vi "Sub Process.vi"(8 "error in (no error)":errorcluster, 11 "MPC_Laser Marked in":refnum<class "MPC_Laser Marked.lvclass">) -> (0 "error out":errorcluster, 3 "MPC_Laser Marked out":refnum<class "MPC_Laser Marked.lvclass">)   [LabVIEW 2019, in "MPC_Laser Marked.lvclass"]
uses:
  MPC_Laser Marked.lvclass
  Main Process Class VI/Ctrl/Flow Action Name.ctl
  Glb/Flow Imform.vi
  LLB/Commonly VI.lvlib
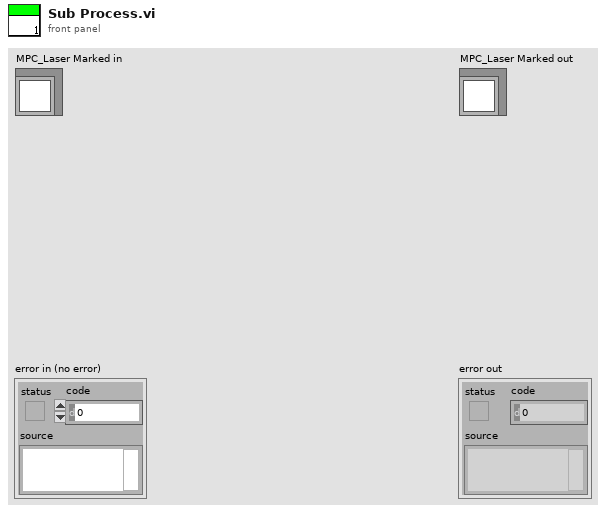
[diagram p1: front panel]
types:
  T1 = typedef "Flow Action Name.ctl" = enum16{"request board", "wait board in", "transfer board in", "imform robot action", "wait robot imform out", "Close Imform Robot", "imform ready out", "wait request", "flow out"}
  T2 = cluster{"AutoRunFlg":refnum<vi>, "Action Finish Flg":refnum<vi>, "Remaining Action":refnum<vi>, "Btn_AutoRun":refnum<vi>, "Manual Flg":refnum<vi>, "Sub Process Error":refnum<vi>}
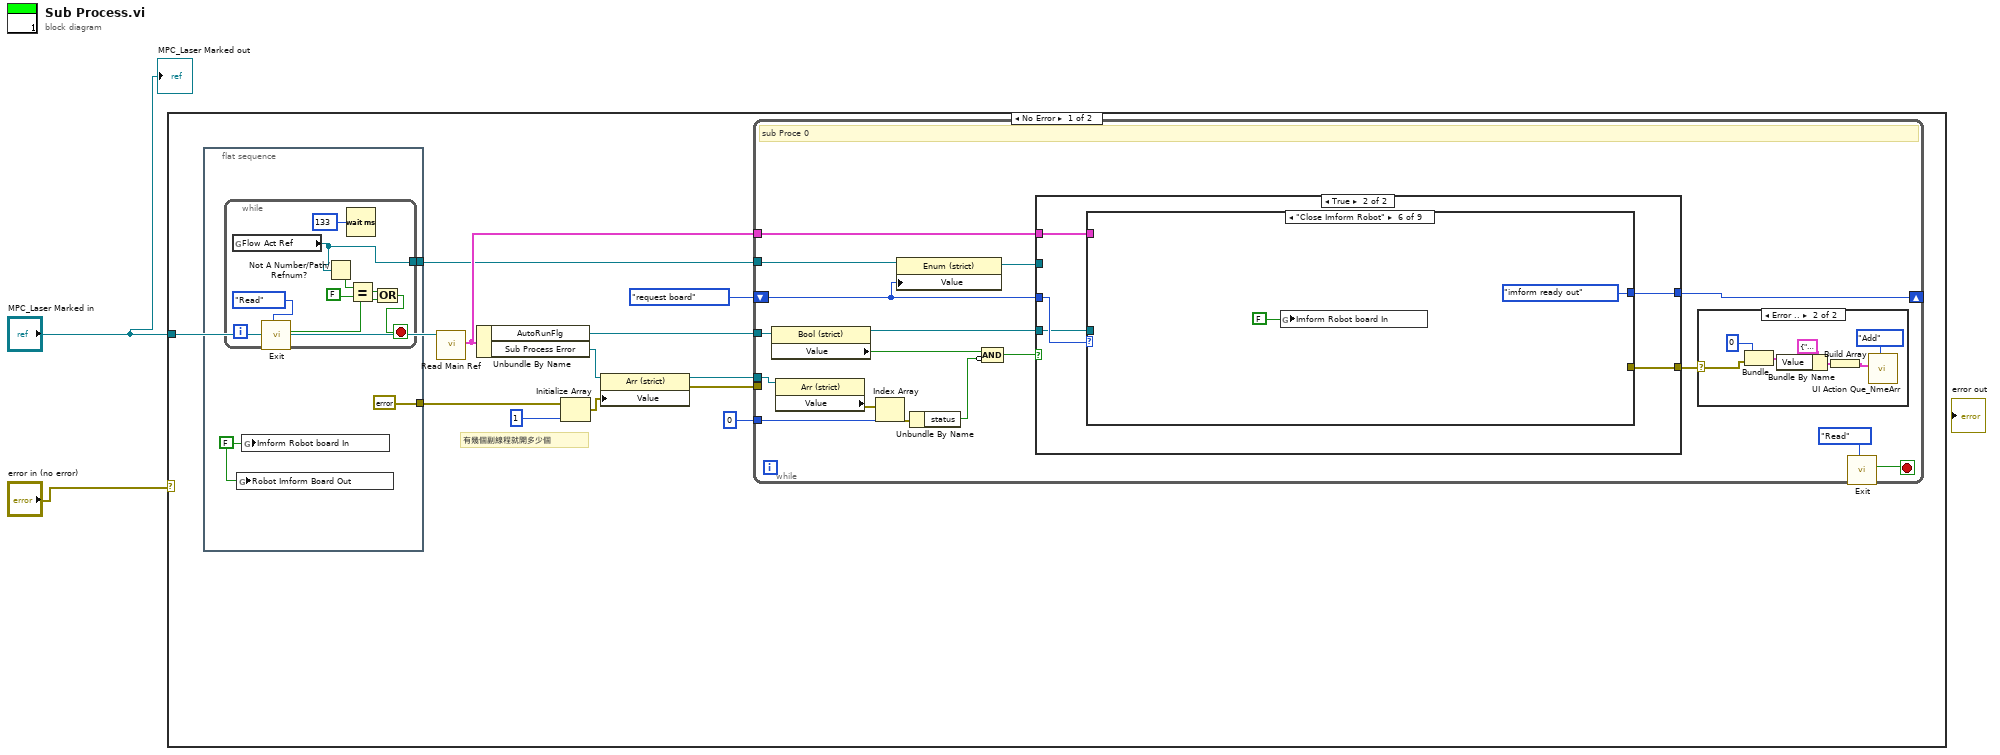
[diagram p0: block diagram]
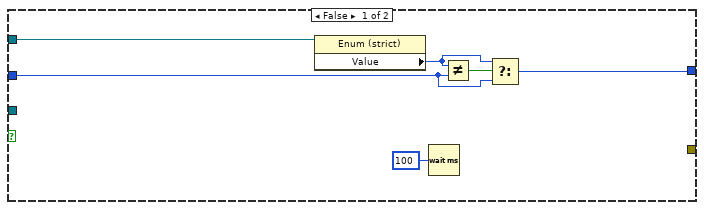
[diagram p3: hidden frame]
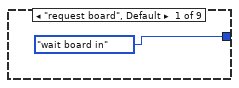
[diagram p4: hidden frame]
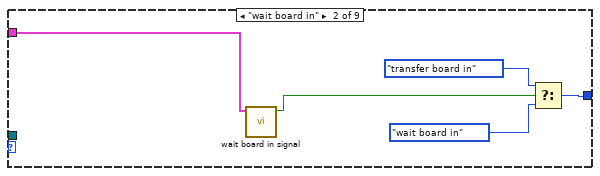
[diagram p5: hidden frame]
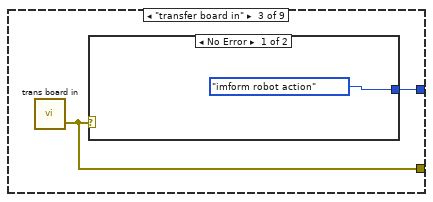
[diagram p6: hidden frame]
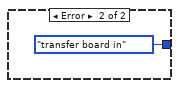
[diagram p7: hidden frame]
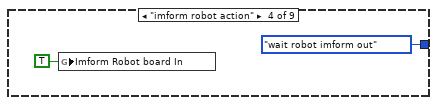
[diagram p8: hidden frame]
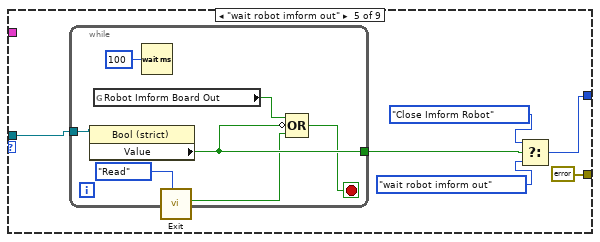
[diagram p9: hidden frame]
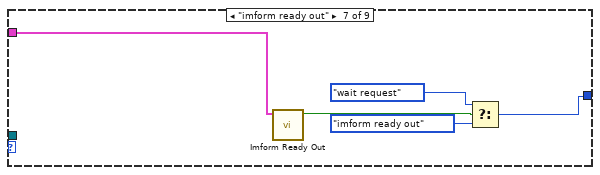
[diagram p10: hidden frame]
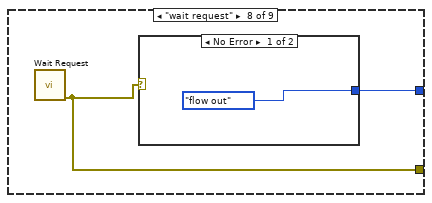
[diagram p11: hidden frame]
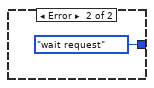
[diagram p12: hidden frame]
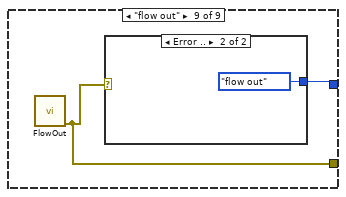
[diagram p13: hidden frame]
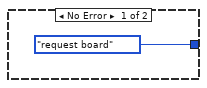
[diagram p14: hidden frame]
diagram:
  n1 = case shown="No Error" "error in (no error)" {
    tunnel: "MPC_Laser Marked in" -> [w14 _]
    frame No Error {
      # "有幾個副線程就開多少個"
      n2 = flat-sequence {
        tunnel: [errorcluster {"status"=FALSE, "code"=0, "source"=""} ("error")] -> w4
        tunnel: [w15] -> w3
        frame #0 {
          w16 = FALSE ("Imform Robot board In")
          n3 = while {
            tunnel: [w24] -> w15
            stop <- w19 stop-if-true
            n4 = global read "Flow Imform.vi" "Flow Act Ref"() -> (w24:refnum<vi>)
            n5 = call "Exit.vi"("Enum"=enum16{"Initial", "Read", "Write"}."Read") -> ("ExitOut"=w20:bool)  [unwired: 10 in]
            n6 = Not A Number/Path/Refnum?(number/path/refnum=w24) -> (NaN/Path/Refnum?=w23:bool)
            n7 = Wait (ms)(milliseconds to wait=u32 133) -> ()  [unwired: 1 out]
            n8 = Equal?(x=w23, y=FALSE ("x")) -> (x = y?=w21:bool)
            n9 = Or(x=w21, y=w20) -> (x .or. y?=w19:bool)
          }
          n10 = global write "Flow Imform.vi" "Robot Imform Board Out"(w16) -> ()
          n11 = global write "Flow Imform.vi" "Imform Robot board In"(w16) -> ()
        }
      }
      n12 = call-dynamic "Read Main Ref.vi"("Main Process Class in"=w14) -> ("Main Ref"=w5:T2)  [unwired: 8 in, 2 out]
      n13 = Unbundle By Name(w5) -> ("AutoRunFlg"=w13:refnum<vi>, "Sub Process Error"=w12:refnum<vi>)
      n14 = Initialize Array(w4, 1 ("dimension size")) -> (w11:errorcluster[])
      n15 = property class="Arr (strict)"(reference=w12, "Value"=w11) -> (reference out=w8:refnum<vi>, error out=w9:errorcluster)  [unwired: 1 in]
      n16 = while {
        tunnel: w13 -> [w42]
        tunnel: w9 -> [_]
        tunnel: w8 -> [w41]
        tunnel: 0 -> [w39]
        shift-right: [w32] -> _
        shift-left: Flow_Action_Name."request board" -> [w34]
        tunnel: w5 -> [w31]
        tunnel: w3 -> [w26]
        stop <- w28 stop-if-true
        # "sub Proce 0"
        n17 = property class="Bool (strict)"(reference=w42) -> (reference out=w29:refnum<vi>, "Value"=w37:bool)  [unwired: 1 in, 1 out]
        n18 = property class="Arr (strict)"(reference=w41) -> ("Value"=w40:errorcluster[])  [unwired: 1 in, 2 out]
        n19 = Index Array(array=w40, index=w39) -> (element=w38:errorcluster)
        n20 = property class="Enum (strict)"(reference=w26, "Value"=w34) -> (reference out=w33:refnum<vi>)  [unwired: 1 in, 1 out]
        n21 = Unbundle By Name(w38) -> ("status"=w36:bool)
        n22 = Compound Arithmetic op=AND(w37, invert w36) -> (w35:bool)
        n23 = case shown="True" w35 {
          tunnel: w34 -> [w51 w60]
          tunnel: w33 -> [w55 _]
          tunnel: [w52 w59] -> w32
          tunnel: w31 -> [_ w58]
          tunnel: [_ w57] -> w30
          tunnel: w29 -> [_ w56]
          frame False {
            n24 = property class="Enum (strict)"(reference=w55) -> ("Value"=w53:T1)  [unwired: 1 in, 2 out]
            n25 = Wait (ms)(milliseconds to wait=u32 100) -> ()  [unwired: 1 out]
            n26 = Not Equal?(x=w53, y=w51) -> (x != y?=w54:bool)
            n27 = Select(t=w53, s=w54, f=w51) -> (s? t:f=w52:T1)
          }
          frame True {
            n28 = case shown="\"Close Imform Robot\"" w60 {
              tunnel: [Flow_Action_Name."wait board in" w62 w68 Flow_Action_Name."wait robot imform out" w75 Flow_Action_Name."imform ready out" w89 w93 w97] -> w59
              tunnel: w58 -> [_ w66 _ _ _ _ w92 _ _]
              tunnel: [_ _ w67 _ errorcluster {"status"=FALSE, "code"=0, "source"=""} ("error out") _ _ w94 w98] -> w57
              tunnel: w56 -> [_ _ _ _ w73 _ _ _ _]
              frame "request board", Default {
              }
              frame "wait board in" {
                n29 = call "wait board in signal.vi"("Main Ref"=w66) -> ("Board Flow in"=w65:bool)  [unwired: 10 in]
                n30 = Select(t=Flow_Action_Name."transfer board in", s=w65, f=Flow_Action_Name."wait board in") -> (s? t:f=w62:T1)
              }
              frame "transfer board in" {
                n31 = call "trans board in.vi"() -> ("error out"=w67:errorcluster)  [unwired: 11 in]
                n32 = case shown="No Error" w67 {
                  tunnel: [Flow_Action_Name."imform robot action" Flow_Action_Name."transfer board in"] -> w68
                  frame No Error {
                  }
                  frame Error {
                  }
                }
              }
              frame "imform robot action" {
                n33 = global write "Flow Imform.vi" "Imform Robot board In"(TRUE ("Imform Robot board In")) -> ()
              }
              frame "wait robot imform out" {
                n34 = while {
                  tunnel: [w82] -> w78
                  tunnel: w73 -> [w79]
                  stop <- w80 stop-if-true
                  n35 = property class="Bool (strict)"(reference=w79) -> ("Value"=w82:bool)  [unwired: 1 in, 2 out]
                  n36 = global read "Flow Imform.vi" "Robot Imform Board Out"() -> (w83:bool)
                  n37 = Wait (ms)(milliseconds to wait=u32 100) -> ()  [unwired: 1 out]
                  n38 = call "Exit.vi"("Enum"=enum16{"Initial", "Read", "Write"}."Read") -> ("ExitOut"=w81:bool)  [unwired: 10 in]
                  n39 = Compound Arithmetic op=OR(w83, invert w82, w81) -> (w80:bool)
                }
                n40 = Select(t=Flow_Action_Name."Close Imform Robot", s=w78, f=Flow_Action_Name."wait robot imform out") -> (s? t:f=w75:T1)
              }
              frame "Close Imform Robot" {
                n41 = global write "Flow Imform.vi" "Imform Robot board In"(FALSE ("Robot Imform Board Out")) -> ()
              }
              frame "imform ready out" {
                n42 = call "Imform Ready Out.vi"("Main Ref"=w92) -> ("Flow Out"=w91:bool)  [unwired: 10 in]
                n43 = Select(t=Flow_Action_Name."wait request", s=w91, f=Flow_Action_Name."imform ready out") -> (s? t:f=w89:T1)
              }
              frame "wait request" {
                n44 = call "Wait Request.vi"() -> ("error out"=w94:errorcluster)  [unwired: 11 in]
                n45 = case shown="No Error" w94 {
                  tunnel: [Flow_Action_Name."flow out" Flow_Action_Name."wait request"] -> w93
                  frame No Error {
                  }
                  frame Error {
                  }
                }
              }
              frame "flow out" {
                n46 = call "FlowOut.vi"() -> ("error out"=w98:errorcluster)  [unwired: 11 in]
                n47 = case shown="Error .." w98 {
                  tunnel: [Flow_Action_Name."request board" Flow_Action_Name."flow out"] -> w97
                  frame No Error {
                  }
                  frame Error {
                  }
                }
              }
            }
          }
        }
        n48 = case shown="Error .." w30 {
          selector: w30 -> [_ w43]
          frame No Error {
          }
          frame Error {
            n49 = Bundle(0, "error IO"=w43) -> (w44:cluster{i32, "error IO":errorcluster})  [unwired: 1 in]
            n50 = Bundle By Name(cluster=cluster{"Action":string, "Value":variant} {"Action"="Updata Sub Error", "Value"=variant} ("UI Action"), "Value"=w44) -> (w47:cluster{"Action":string, "Value":variant})
            n51 = Build Array(w47) -> (w46:cluster{"Action":string, "Value":variant}[])
            n52 = call "UI Action Que_NmeArr.vi"("Action"=enum16{"Initial", "Add", "Release"}."Add", "UI Process"=w46) -> ()  [unwired: 8 in, 2 out]
          }
        }
        n53 = call "Exit.vi"("Enum"=enum16{"Initial", "Read", "Write"}."Read") -> ("ExitOut"=w28:bool)  [unwired: 10 in]
      }
    }
    frame Error {
    }
  }
  "MPC_Laser Marked out" <- "MPC_Laser Marked in"
